vi "Launcher.vi"() -> ()   [LabVIEW 2025]
uses:
  <vilib>/Utility/error.llb/DialogType.ctl
  Full User Interface/Full User Interface.lvlib
panel:
  out "Status":string
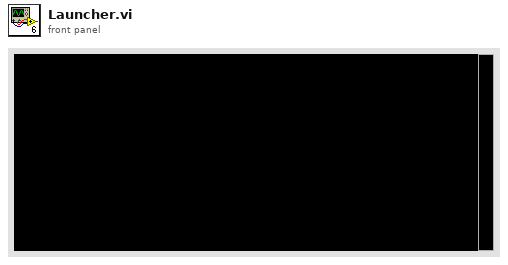
[diagram p1: front panel]
types:
  T1 = enum32{"Invalid", "Standard", "Closed", "Hidden", "Minimized", "Maximized"}
  T2 = typedef "Full User Interface.lvlib/Broadcast Events--cluster.ctl" = cluster{"Module Did Init":refnum<user-event>, "Status Updated":refnum<user-event>, "Error Reported":refnum<user-event>, "Module Did Stop":refnum<user-event>, "Update Module Execution Status":refnum<user-event>}
  T3 = typedef "DialogType.ctl" = u16
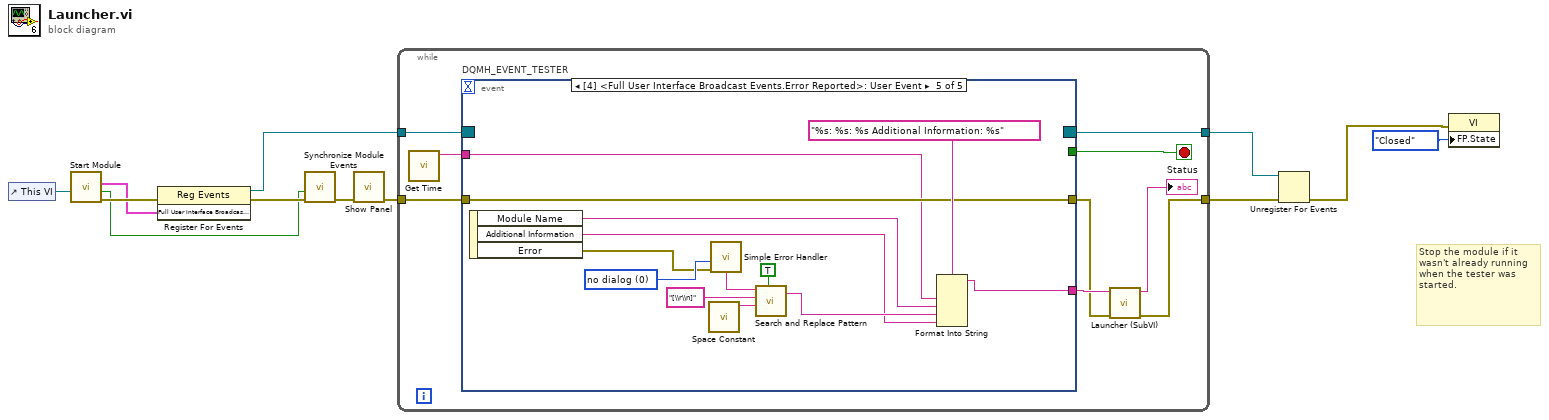
[diagram p0: block diagram]
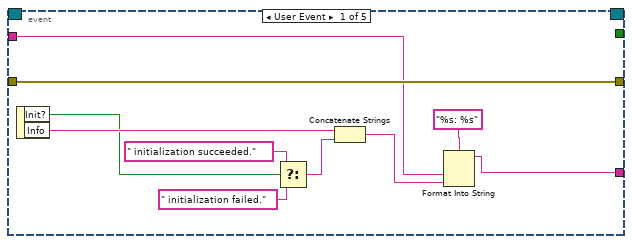
[diagram p2: hidden frame]
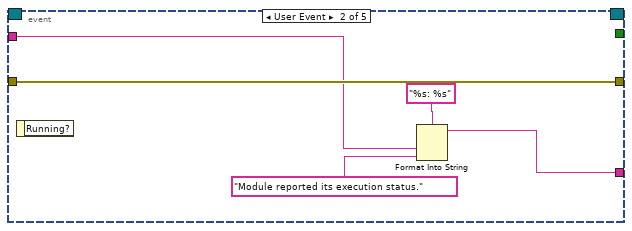
[diagram p3: hidden frame]
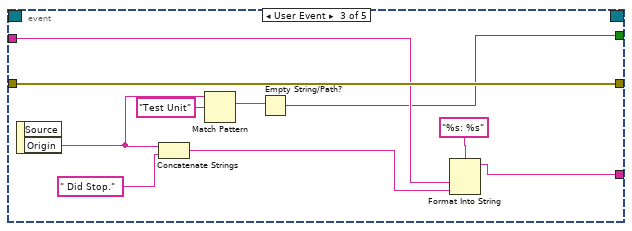
[diagram p4: hidden frame]
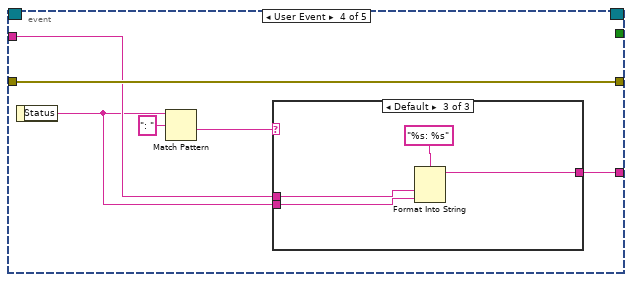
[diagram p5: hidden frame]
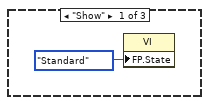
[diagram p6: hidden frame]
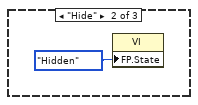
[diagram p7: hidden frame]
diagram:
  # "Stop the module if it wasn't already running when the tester was started."
  n1 = control-ref of="This VI"() -> (w1:refnum<vi>)
  n2 = call "Start Module.vi"("VI"=w1) -> ("error out"=w9:errorcluster, "Wait for Event Sync?"=w8:bool, "Full User Interface Broadcast Events"=w7:T2)  [unwired: 7 in, 1 out]
  n3 = register-events(error in=w9, w7) -> (reference out=w5:refnum<event-registration>, error out=w10:errorcluster)  [unwired: 1 in]
  n4 = call "Synchronize Module Events.vi"("error in"=w10, "Wait for Event Sync?"=w8) -> ("error out"=w6:errorcluster)  [unwired: 9 in]
  n5 = call "Show Panel.vi"("error in"=w6) -> ("error out"=w4:errorcluster)  [unwired: 10 in]
  n6 = while {
    tunnel: w5 -> [w21]
    tunnel: [w13] -> w11
    tunnel: w4 -> [w20]
    tunnel: [w19] -> w12
    stop <- w18 stop-if-true
    n7 = call "Get Time.vi"() -> ("time"=w17:string)  [unwired: 11 in]
    n8 = event "DQMH_EVENT_TESTER" shown="[4] <Full User Interface Broadcast Events.Error Reported>: User Event" {
      selector: w21 -> [_ _ _ _ _]
      dyn-events: [_ _ _ _ _] -> w19
      timeout: _ -> [_ _ _ _ _]
      tunnel: [_ _ w38 _ _] -> w18
      tunnel: [w31 w34 w43 w52 w64] -> w14
      tunnel: w20 -> [w31 w34 w43 w52 w64]
      tunnel: w17 -> [w23 w33 w42 w51 w60]
      tunnel: [w22 w32 w37 w47 w59] -> w15
      event User Event {
        n9 = event-data() -> ("Init?"=w27:bool, "Info"=w29:string)  [unwired: 1 in]
        n10 = Select(t=" initialization succeeded.", s=w27, f=" initialization failed.") -> (s? t:f=w24:string)
        n11 = Concatenate Strings(w29, w24) -> (w28:string)
        n12 = Format Into String(format string="%s: %s", w23, w28) -> (resulting string=w22:string)  [unwired: 2 in, 1 out]
      }
      event User Event {
        n13 = event-data() -> ()  [unwired: 1 in, 1 out]
        n14 = Format Into String(format string="%s: %s", w33, "Module reported its execution status.") -> (resulting string=w32:string)  [unwired: 2 in, 1 out]
      }
      event User Event {
        n15 = event-data() -> ("Origin"=w41:string)  [unwired: 1 in, 1 out]
        n16 = Concatenate Strings(w41, " Did Stop.") -> (w45:string)
        n17 = Match Pattern(string=w41, regular expression="Test Unit") -> (match substring=w39:string)  [unwired: 1 in, 3 out]
        n18 = Empty String/Path?(string/path=w39) -> (empty?=w38:bool)
        n19 = Format Into String(format string="%s: %s", w42, w45) -> (resulting string=w37:string)  [unwired: 2 in, 1 out]
      }
      event User Event {
        n20 = event-data() -> ("Status"=w50:string)  [unwired: 1 in]
        n21 = Match Pattern(string=w50, regular expression=": ") -> (after substring=w48:string)  [unwired: 1 in, 3 out]
        n22 = case shown="Default" w48 {
          tunnel: w51 -> [_ _ w57]
          tunnel: w50 -> [_ _ w56]
          tunnel: [_ _ w55] -> w47
          frame "Show" {
            n23 = property class="VI"("FP.State"=T1."Standard" ("Front Panel Window:State")) -> ()  [unwired: 2 in, 2 out]
          }
          frame "Hide" {
            n24 = property class="VI"("FP.State"=T1."Hidden" ("Front Panel Window:State")) -> ()  [unwired: 2 in, 2 out]
          }
          frame Default {
            n25 = Format Into String(format string="%s: %s", w57, w56) -> (resulting string=w55:string)  [unwired: 2 in, 1 out]
          }
        }
      }
      event User Event {
        w65 = T3 0 items=["no dialog", "OK message", "continue or stop message", "OK message + warnings", "continue/stop + warnings"] ("type of dialog (OK msg:1)")
        n26 = event-data() -> ("Module Name"=w63:string, "Additional Information"=w62:string, "Error"=w61:errorcluster)  [unwired: 1 in]
        n27 = call <vilib>:"Space Constant.vi"() -> ("String"=w69:string)
        n28 = call <vilib>:"Simple Error Handler.vi"("type of dialog (OK msg:1)"=w65, "error in (no error)"=w61) -> ("message"=w66:string)  [unwired: 3 in, 4 out]
        n29 = call <vilib>:"Search and Replace Pattern.vi"("string"=w66, "regular expression (\"\")"="[\\r\\n]" ("regular expression (\"\")"), "replace string (\"\")"=w69, "replace all? (F)"=TRUE ("replace all CR/LF with spaces")) -> ("result string"=w67:string)  [unwired: 1 in, 1 out]
        n30 = Format Into String(format string="%s: %s: %s Additional Information: %s", w60, w63, w67, w62) -> (resulting string=w59:string)  [unwired: 2 in, 1 out]
      }
    }
    n31 = call "Launcher (SubVI).vi"("error in (no error)"=w14, "String"=w15) -> ("error out"=w13:errorcluster, "spreadsheet string"=→"Status":string)  [unwired: 8 in]
  }
  n32 = Unregister For Events(event registration refnum=w12, error in=w11) -> (error out=w2:errorcluster)
  n33 = property class="VI"(error in=w2, "FP.State"=T1."Closed" ("Front Panel Window:State")) -> ()  [unwired: 1 in, 2 out]
